vi "Track.vi"(0 "Power":dbl, 5 "Heading":dbl, 7 "Kp":dbl, 9 "Ramp_L":dbl, 11 "Ramp_R":dbl) -> (4 "Error":dbl, 6 "On Target":bool)   [LabVIEW 2017]
uses:
  <vilib>/addons/control/pid/NI_PID_pid.lvlib
  <vilib>/addons/control/pid/pid.llb/PID (DBL).vi
  <vilib>/Rock Robotics/WPI/ThirdParty/Phoenix-LabVIEW/Pigeon IMU/CTRE_PigeonIMU_GetYPR.vi
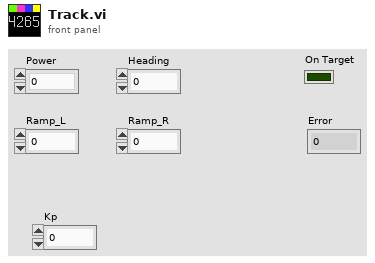
[diagram p1: front panel]
types:
  T1 = typedef "WPI_MotorControlDeviceRef.ctl" = cluster{"DeviceStatus":errorcluster, "Type":T2, "PWM":cluster{"PWM Channel":T3, "DeadBand":T4}, "CAN":cluster{"Device Number":u8, "SetOutput VI Ref":variant, "GetOutput VI Ref":variant, "Enable VI Ref":variant, "Disable VI Ref":variant, "Data":variant}, "Invert":bool, "DIO PWM":cluster{"PWM \"Enable\" Channel":T3, "DIOChannel":T5, "PWM Rate":dbl}}
  T2 = typedef "WPI_MotorControlType.ctl" = enum16{"PWM", "CAN", "DIO PWM"}
  T3 = typedef "FPGA_DIOPWMChannel.ctl" = enum8{"PWM 0", "PWM 1", "PWM 2", "PWM 3", "PWM 4", "PWM 5", "PWM 6", "PWM 7", "PWM 8", "PWM 9", "PWM MXP 0", "PWM MXP 1", "PWM MXP 2", "PWM MXP 3", "PWM MXP 4", "PWM MXP 5", "PWM MXP 6", "PWM MXP 7", "PWM MXP 8", "PWM MXP 9", "Invalid"}
  T4 = typedef "WPI_PWMDeadband.ctl" = cluster{"Name":string, "maxPositivePwm":i32, "minPositivePwm":i32, "centerPwm":i32, "maxNegativePwm":i32, "minNegativePwm":i32, "angularRange":u16}
  T5 = typedef "FPGA_DIOChannel.ctl" = enum8{"DIO 0", "DIO 1", "DIO 2", "DIO 3", "DIO 4", "DIO 5", "DIO 6", "DIO 7", "DIO 8", "DIO 9", "DIO MXP 0", "DIO MXP 1", "DIO MXP 2", "DIO MXP 3", "DIO MXP 4", "DIO MXP 5", "DIO MXP 6", "DIO MXP 7", "DIO MXP 8", "DIO MXP 9", "DIO MXP 10", "DIO MXP 11", "DIO MXP 12", "DIO MXP 13", "DIO MXP 14", "DIO MXP 15", "SPI Port CS1", "SPI Port CS2", "SPI Port CS3", "SPI Port MISO", "SPI Port MOSI", "Invalid"}
  T6 = typedef "CTRE_PigeonIMU_DeviceRef.ctl" = cluster{"DeviceStatus":errorcluster, "Device Number":u8, "Type":T7, "Device ID":u32, "Handle":u64, "UsageFrame":u32, "Library Path":path}
  T7 = typedef "CTRE_PigeonIMU_ConnectionType.ctl" = u32
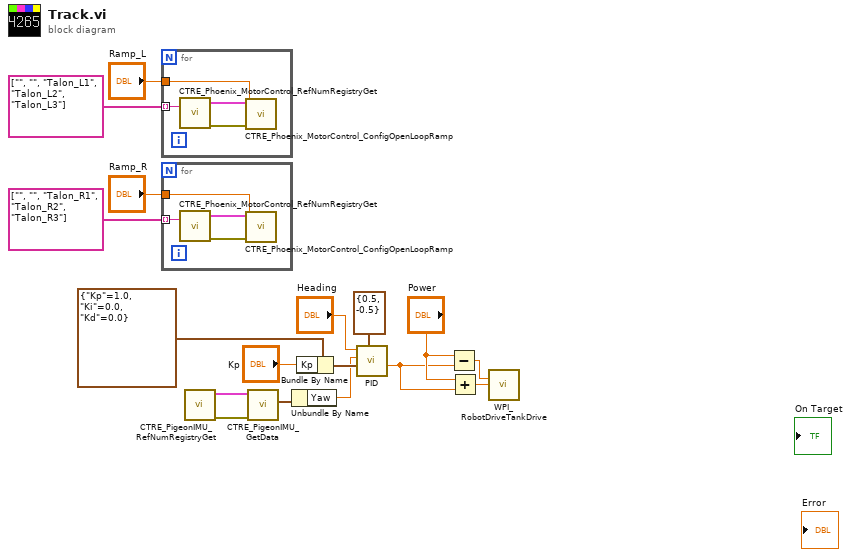
[diagram p0: block diagram]
diagram:
  n1 = for {
    tunnel: "Ramp_L" -> [w19]
    tunnel: string[] ["", "", "Talon_L1", "Talon_L2", "Talon_L3"] -> [w18] mode=indexing
    n2 = call <vilib>:"CTRE_Phoenix_MotorControl_RefNumRegistryGet.vi"("refnum name"=w18) -> ("error out"=w21:errorcluster, "PhoenixMotorControlDevRef"=w20:T1)  [unwired: 9 in]
    n3 = call <vilib>:"CTRE_Phoenix_MotorControl_ConfigOpenLoopRamp.vi"("error in (no error)"=w21, "secondsFromNeutralToFull"=w19, "PhoenixMotorControlDevRef"=w20) -> ()  [unwired: 7 in, 2 out]
  }
  n4 = for {
    tunnel: "Ramp_R" -> [w23]
    tunnel: string[] ["", "", "Talon_R1", "Talon_R2", "Talon_R3"] -> [w22] mode=indexing
    n5 = call <vilib>:"CTRE_Phoenix_MotorControl_RefNumRegistryGet.vi"("refnum name"=w22) -> ("error out"=w25:errorcluster, "PhoenixMotorControlDevRef"=w24:T1)  [unwired: 9 in]
    n6 = call <vilib>:"CTRE_Phoenix_MotorControl_ConfigOpenLoopRamp.vi"("error in (no error)"=w25, "secondsFromNeutralToFull"=w23, "PhoenixMotorControlDevRef"=w24) -> ()  [unwired: 7 in, 2 out]
  }
  n7 = call <vilib>:"CTRE_PigeonIMU_RefNumRegistryGet.vi"() -> ("error out"=w11:errorcluster, "PigeonIMUDevRef"=w12:T6)  [unwired: 10 in]
  n8 = call-poly <vilib>:"CTRE_PigeonIMU_GetData.vi"("error in (no error)"=w11, "PigeonIMUDevRef"=w12) -> ("Yaw Pitch Roll"=w6:cluster{"Yaw":dbl, "Pitch":dbl, "Roll":dbl})  [unwired: 7 in, 2 out]
  n9 = Unbundle By Name(w6) -> ("Yaw"=w5:dbl)
  n10 = Bundle By Name(cluster=cluster{"Kp":dbl, "Ki":dbl, "Kd":dbl} {"Kp"=1.0, "Ki"=0.0, "Kd"=0.0}, "Kp"="Kp") -> (w16:cluster{"Kp":dbl, "Ki":dbl, "Kd":dbl})
  n11 = call-poly <vilib>:"PID.vi"("output range"=cluster{"output high":dbl, "output low":dbl} {"output high"=0.5, "output low"=-0.5}, "PID gains"=w16, "process variable"=w5, "setpoint"="Heading") -> ("output"=w7:dbl)  [unwired: 6 in, 1 out]
  n12 = Subtract(x="Power", y=w7) -> (x-y=w9:dbl)
  n13 = Add(x="Power", y=w7) -> (x+y=w10:dbl)
  n14 = call <vilib>:"WPI_RobotDriveTankDrive.vi"("Right axis value"=w10, "Left axis value"=w9) -> ()  [unwired: 7 in, 3 out]
